vi "WolframAlpha.vi"() -> ()   [LabVIEW 2020]
uses:
  <vilib>/httpClient/LabVIEWHTTPClient.lvlib
panel:
  out "body":string
  out "headers":string
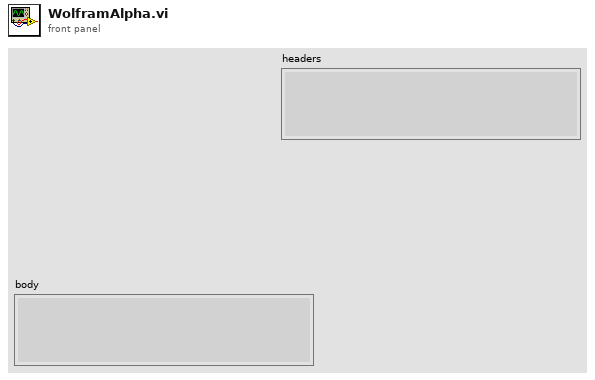
[diagram p1: front panel]
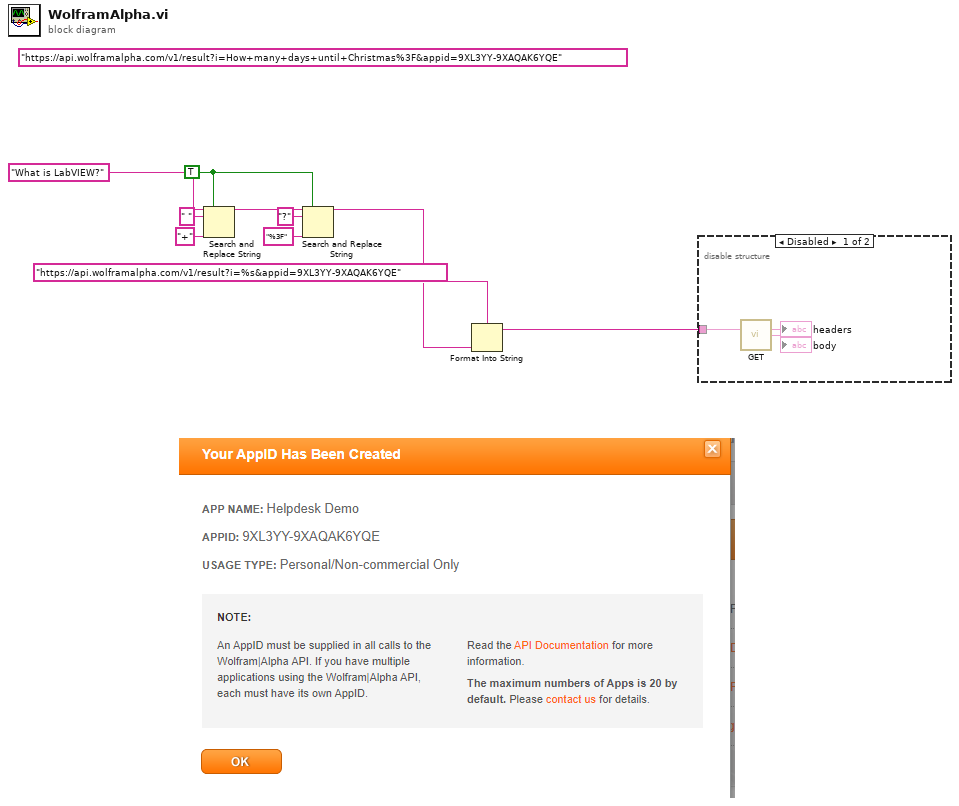
[diagram p0: block diagram]
diagram:
  (unwired) "https://api.wolframalpha.com/v1/result?i=How+many+days+until+Christmas%3F&appid=9XL3YY-9XAQAK6YQE" ("url")
  w2 = TRUE ("ignore case? (F)")
  n1 = Search and Replace String(replace all?=w2, input string="What is LabVIEW?" ("unescaped string in"), search string=" ", replace string="+" ("replace string (\"\")")) -> (result string=w6:string)  [unwired: 4 in, 3 out]
  n2 = Search and Replace String(replace all?=w2, input string=w6, search string="?", replace string="%3F" ("replace string (\"\")")) -> (result string=w3:string)  [unwired: 4 in, 3 out]
  n3 = Format Into String(format string="https://api.wolframalpha.com/v1/result?i=%s&appid=9XL3YY-9XAQAK6YQE" ("url"), w3) -> (resulting string=w1:string)  [unwired: 2 in, 1 out]
  n4 = disable-structure shown="Disabled" {
    disable-tunnel: w1 -> [w11 _]
    frame Disabled {
      n5 = call <vilib>:"GET.vi"("url"=w11) -> ("headers"=→"headers":string, "body"=→"body":string)  [unwired: 11 in, 2 out]
    }
    frame Enabled {
    }
  }
